vi "init runtime data structures.vi"(4 "write directory":path, 6 "read directory":path, 8 "error in":errorcluster, 9 "data allocations":T3, 10 "lines":T1[](array[typedef]), 11 "shared memory module runtime in":refnum<class "Shared Memory Runtime.lvclass">) -> (0 "error out":errorcluster, 3 "shared memory module runtime out":refnum<class "Shared Memory Runtime.lvclass">)   [LabVIEW 2013, in "Shared Memory Runtime.lvclass"]
uses:
  Shared Memory Runtime.lvclass
  <vilib>/NI/Tag Bus Module Framework/channel/data tables.ctl
  <vilib>/NI/Tag Bus/dictionary/data dictionary.lvclass
  <vilib>/NI/Tag Bus/dictionary table pair.ctl
  <vilib>/NI/Tag Bus/table/data table.ctl
  configuration/line configuration.ctl
  <vilib>/NI/Tag Bus Module Framework/channel/TBM channel.lvclass
  <vilib>/NI/Tag Bus/tag/Data Type.ctl
  <vilib>/NI/Tag Bus Module Framework/channel/channel classification.ctl
  <vilib>/NI/Tag Bus Module Framework/channel/TBM channel.lvclass/TBM channel.ctl
  <vilib>/NI/Tag Bus/tag/tag descriptor.lvclass/tag descriptor.ctl
  Shared Memory Runtime.lvclass/Shared Memory Runtime.ctl
  shared memory module runtime.ctl
  <vilib>/NI/Tag Bus/tag/read tag name.vi
  <vilib>/NI/Tag Bus/dictionary/locate tag.vi
  <vilib>/NI/Tag Bus/tag/tag descriptor.lvclass
  <vilib>/NI/Tag Bus/table/data table.lvlib
  <vilib>/NI/Tag Bus/tag bus.lvlib
  configuration/Shared Memory Configuration.lvclass
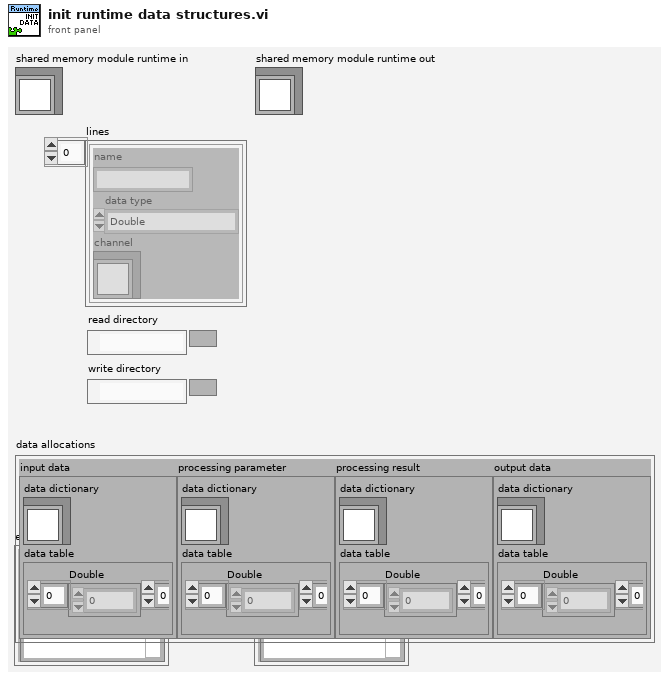
[diagram p1: front panel]
types:
  T1 = typedef "Shared Memory Configuration.lvclass/line configuration.ctl" = cluster{"name":string, "data type":T2, "channel":refnum<class "TBM channel.lvclass">}
  T2 = typedef "tag bus.lvlib/tag descriptor.lvclass/Data Type.ctl" = enum16{"Double", "Single", "I64", "I32", "I16", "I8", "U64", "U32", "U16", "U8", "Boolean", "String", "Array of Double", "Array of Single", "Array of I64", "Array of I32", "Array of I16", "Array of I8", "Array of U64", "Array of U32", "Array of U16", "Array of U8", "Array of Boolean", "Array of String"}
  T3 = typedef "TBM channel.lvclass/data tables.ctl" = cluster{"input data":T4, "processing parameter":T4, "processing result":T4, "output data":T4}
  T4 = typedef "tag bus.lvlib/dictionary table pair.ctl" = cluster{"data dictionary":refnum<class "data dictionary.lvclass">, "data table":T5}
  T5 = typedef "tag bus.lvlib/data table.lvlib/data table.ctl" = cluster{"Double":dbl[], "Single":sgl[], "I64":i64[], "I32":i32[], "I16":i16[], "I8":i8[], "U64":u64[], "U32":u32[], "U16":u16[], "U8":u8[], "Boolean":bool[], "String":string[], "Array of Double":cluster{"DBL Array":dbl[]}[], "Array of Single":cluster{"SGL Array":sgl[]}[], "Array of I64":cluster{"I64 Array":i64[]}[], "Array of I32":cluster{"I32 Array":i32[]}[], "Array of I16":cluster{"I16 Array":i16[]}[], "Array of I8":cluster{"I8 Array":i8[]}[], "Array of U64":cluster{"U64 Array":u64[]}[], "Array of U32":cluster{"U32 Array":u32[]}[], "Array of U16":cluster{"U16 Array":u16[]}[], "Array of U8":cluster{"U8 Array":u8[]}[], "Array of Boolean":cluster{"Boolean Array":bool[]}[], "Array of String":cluster{"String Array":string[]}[]}
  T6 = typedef "TBM channel.lvclass/channel classification.ctl" = enum16{"input data", "output data", "processing parameter", "processing result"}
  T7 = enum16{"open", "replace", "create", "open or create", "replace or create", "replace or create with confirmation"}
  T8 = typedef "Shared Memory Runtime.lvclass/shared memory module runtime.ctl" = cluster{"refnum":refnum<file>, "name":string, "data type":T2, "number of tags":i32, "indices":cluster{"index":i32[]}, "data array":cluster{"data":dbl[]}, "file array":cluster{"data":dbl[]}}
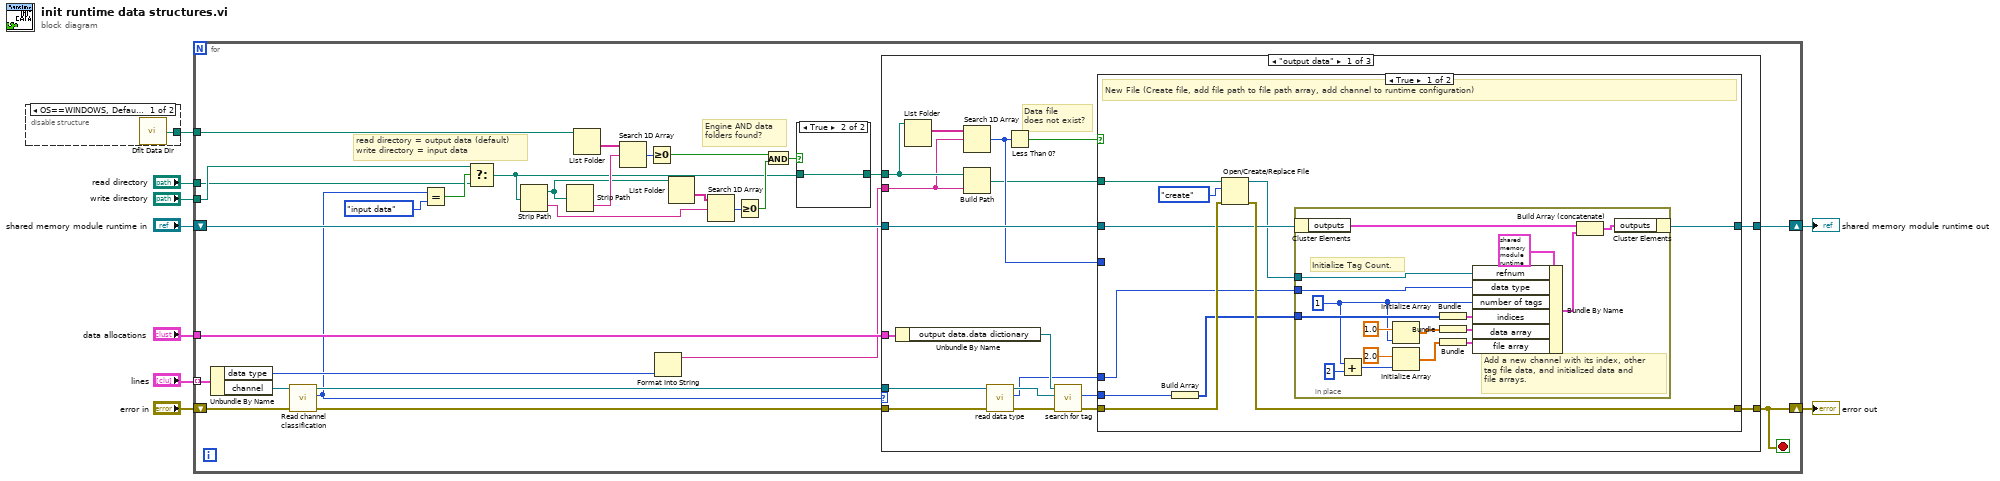
[diagram p0: block diagram]
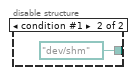
[diagram p2: hidden frame]
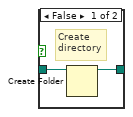
[diagram p3: hidden frame]
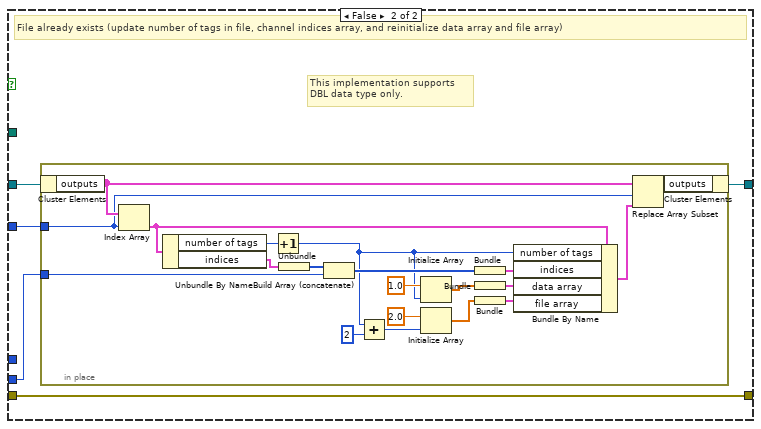
[diagram p4: hidden frame]
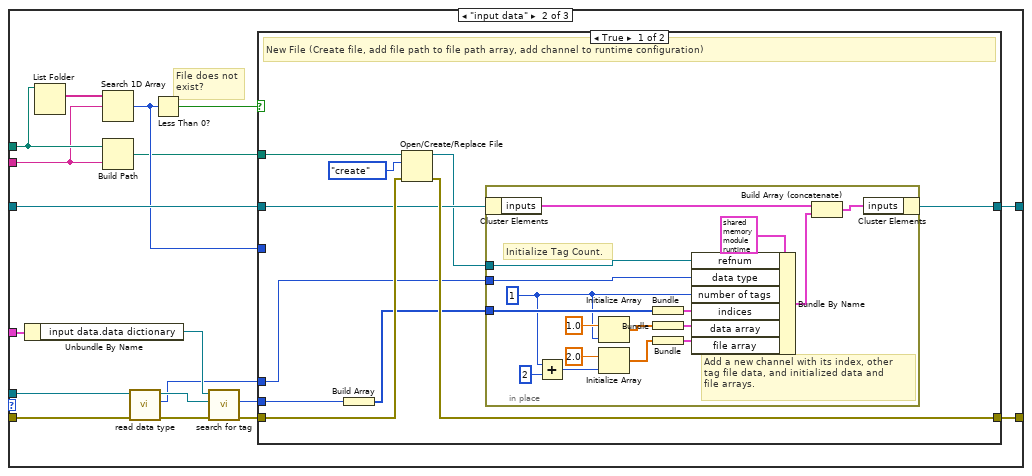
[diagram p5: hidden frame]
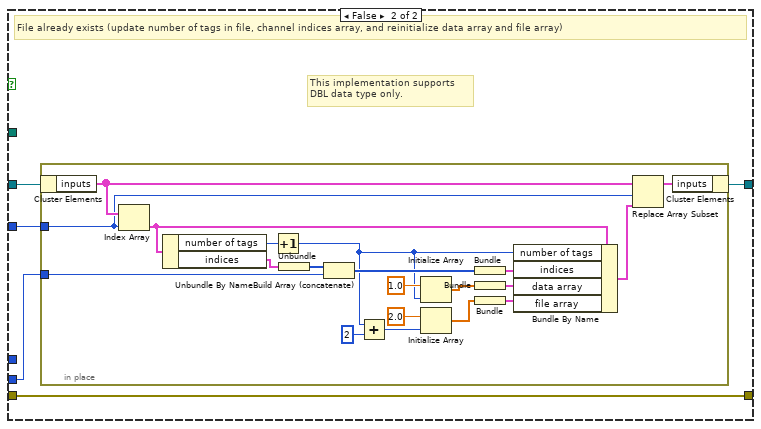
[diagram p6: hidden frame]
diagram:
  n1 = disable-structure shown="OS==WINDOWS, Default" {
    disable-tunnel: [w10 path "/dev/shm"] -> w3
    frame condition #0 (active) {
      n2 = call <vilib>:"Dflt Data Dir.vi"() -> ("App:Default Data Directory"=w10:path)
    }
    frame condition #1 {
    }
  }
  n3 = for {
    shift-right: [w40] -> w8
    shift-left: "error in" -> [w37]
    tunnel: "lines" -> [w38] mode=indexing
    tunnel: "data allocations" -> [w39]
    tunnel: w3 -> [w26]
    shift-right: [w32] -> w4
    shift-left: "shared memory module runtime in" -> [w33]
    tunnel: "read directory" -> [w12]
    tunnel: "write directory" -> [w13]
    stop <- w40 stop-if-true
    # "read directory = output data (default)\nwrite directory = input data"
    # "Engine AND data \nfolders found?"
    n4 = Unbundle By Name(w38) -> ("data type"=w31:T2, "channel"=w35:refnum<class "TBM channel.lvclass">)
    n5 = call <vilib>:"Read channel classification.vi"("error in"=w37, "channel in"=w35) -> ("error out"=w36:errorcluster, "channel classification"=w17:T6, "channel out"=w34:refnum<class "TBM channel.lvclass">)  [unwired: 7 in]
    n6 = Equal?(x=w17, y=channel_classification."input data") -> (x = y?=w15:bool)
    n7 = Select(t=w13, s=w15, f=w12) -> (s? t:f=w14:path)
    n8 = Strip Path(path=w14) -> (stripped path=w21:path, name=w19:string)
    n9 = Strip Path(path=w21) -> (name=w27:string)  [unwired: 1 out]
    n10 = List Folder(path=w26) -> (folder names=w29:string[])  [unwired: 3 in, 3 out]
    n11 = Search 1D Array(1D array=w29, element=w27) -> (index of element=w28:i32)  [unwired: 1 in]
    n12 = Greater Or Equal To 0?(x=w28) -> (x >= 0?=w24:bool)
    n13 = Format Into String(w31) -> (resulting string=w18:string)  [unwired: 3 in, 1 out]
    n14 = List Folder(path=w21) -> (folder names=w20:string[])  [unwired: 3 in, 3 out]
    n15 = Search 1D Array(1D array=w20, element=w19) -> (index of element=w25:i32)  [unwired: 1 in]
    n16 = Greater Or Equal To 0?(x=w25) -> (x >= 0?=w23:bool)
    n17 = And(x=w24, y=w23) -> (x .and. y?=w22:bool)
    n18 = case shown="True" w22 {
      tunnel: [w41 w43] -> w30
      tunnel: w14 -> [w42 w43]
      frame False {
        # "Create\ndirectory"
        n19 = Create Folder(path (use dialog)=w42) -> (created path=w41:path)  [unwired: 2 in, 2 out]
      }
      frame True {
      }
    }
    n20 = case shown="\"output data\"" w17 {
      tunnel: [w53 w123 w185] -> w40
      tunnel: w36 -> [w60 w130 w185]
      tunnel: w39 -> [w58 w128 _]
      tunnel: w34 -> [w56 w126 _]
      tunnel: w30 -> [w46 w116 _]
      tunnel: w18 -> [w45 w115 _]
      tunnel: w33 -> [w51 w121 w184]
      tunnel: [w50 w120 w184] -> w32
      frame "output data" {
        # "Data file \ndoes not exist?"
        n21 = Unbundle By Name(w58) -> ("output data.data dictionary"=w57:refnum<class "data dictionary.lvclass">)
        n22 = List Folder(path=w46) -> (filenames=w47:string[])  [unwired: 3 in, 3 out]
        n23 = Search 1D Array(1D array=w47, element=w45) -> (index of element=w49:i32)  [unwired: 1 in]
        n24 = Build Path(base path=w46, name or relative path=w45) -> (appended path=w44:path)
        n25 = call <vilib>:"read data type.vi"("error in"=w60, "system tag in"=w56) -> ("error out"=w59:errorcluster, "data type"=w54:T2, "system tag out"=w61:refnum<class "TBM channel.lvclass">)  [unwired: 7 in]
        n26 = Less Than 0?(x=w49) -> (x < 0?=w52:bool)
        n27 = call <vilib>:"search for tag.vi"("error in"=w59, "system tag"=w61, "data dictionary in"=w57) -> ("error out"=w55:errorcluster, "index"=w48:i32)  [unwired: 6 in, 1 out]
        n28 = case shown="True" w52 {
          tunnel: w44 -> [w69 _]
          tunnel: w55 -> [w71 w93]
          tunnel: w54 -> [w64 _]
          tunnel: [w70 w93] -> w53
          tunnel: w51 -> [w67 w92]
          tunnel: [w66 w90] -> w50
          tunnel: w49 -> [_ w91]
          tunnel: w48 -> [w63 w89]
          frame True {
            # "New File (Create file, add file path to file path array, add channel to runtime configuration)"
            n29 = Build Array(w63) -> (w62:i32[])
            n30 = Open/Create/Replace File(file path (use dialog)=w69, error in=w71, operation (0:open)=T7."create") -> (refnum out=w65:refnum<file>, error out=w70:errorcluster)  [unwired: 3 in, 1 out]
            n31 = in-place {
              in-place-border: w62 -> [w88]
              in-place-border: w65 -> [w78]
              in-place-border: w64 -> [w77]
              w72 = 1 ("y")
              # "Initialize Tag Count."
              # "Add a new channel with its index, other \ntag file data, and initialized data and \nfile arrays."
              n32 = in-place-cluster #1(w67) -> ("outputs"=w76:T8[])
              n33 = Add(x=w72, y=2) -> (x+y=w79:i32)
              n34 = Initialize Array(1.0 ("element"), w72) -> (w84:dbl[])
              n35 = Initialize Array(2.0 ("element"), w79) -> (w82:dbl[])
              n36 = Bundle(w88) -> (w87:cluster{i32[]})  [unwired: 1 in]
              n37 = Bundle(w84) -> (w83:cluster{dbl[]})  [unwired: 1 in]
              n38 = Bundle(w82) -> (w81:cluster{dbl[]})  [unwired: 1 in]
              n39 = Bundle By Name(cluster=T8 {"refnum"=refnum, "name"="", "data type"=enum."Double", "number of tags"=0, "indices"={"index"=[]}, "data array"={"data"=[]}, "file array"={"data"=[]}} ("tag config"), "refnum"=w78, "data type"=w77, "number of tags"=w72, "indices"=w87, "data array"=w83, "file array"=w81) -> (w73:T8)
              n40 = Build Array (concatenate)(w76, w73) -> (w75:T8[])
              n41 = in-place-cluster #1("outputs"=w75) -> (w66:refnum<class "Shared Memory Runtime.lvclass">)
            }
          }
          frame False {
            # "This implementation supports \nDBL data type only."
            # "File already exists (update number of tags in file, channel indices array, and reinitialize data array and file array)"
            n42 = in-place {
              in-place-border: w91 -> [w101]
              in-place-border: w89 -> [w97]
              n43 = in-place-cluster #2(w92) -> ("outputs"=w104:T8[])
              n44 = Index Array(array=w104, index=w101) -> (element=w100:T8)
              n45 = Unbundle By Name(w100) -> ("number of tags"=w95:i32, "indices"=w99:cluster{"index":i32[]})
              n46 = Increment(x=w95) -> (x+1=w94:i32)
              n47 = Unbundle(w99) -> ("index"=w98:i32[])
              n48 = Build Array (concatenate)(w98, w97) -> (w96:i32[])
              n49 = Add(x=w94, y=2) -> (x+y=w105:i32)
              n50 = Initialize Array(1.0 ("element"), w94) -> (w110:dbl[])
              n51 = Initialize Array(2.0 ("element"), w105) -> (w108:dbl[])
              n52 = Bundle(w96) -> (w113:cluster{i32[]})  [unwired: 1 in]
              n53 = Bundle(w110) -> (w109:cluster{dbl[]})  [unwired: 1 in]
              n54 = Bundle(w108) -> (w107:cluster{dbl[]})  [unwired: 1 in]
              n55 = Bundle By Name(cluster=w100, "number of tags"=w94, "indices"=w113, "data array"=w109, "file array"=w107) -> (w102:T8)
              n56 = Replace Array Subset(array=w104, new element=w102, index=w101) -> (w103:T8[])
              n57 = in-place-cluster #2("outputs"=w103) -> (w90:refnum<class "Shared Memory Runtime.lvclass">)
            }
          }
        }
      }
      frame "input data" {
        # "File does not\nexist?"
        n58 = Unbundle By Name(w128) -> ("input data.data dictionary"=w127:refnum<class "data dictionary.lvclass">)
        n59 = List Folder(path=w116) -> (filenames=w117:string[])  [unwired: 3 in, 3 out]
        n60 = Search 1D Array(1D array=w117, element=w115) -> (index of element=w119:i32)  [unwired: 1 in]
        n61 = Build Path(base path=w116, name or relative path=w115) -> (appended path=w114:path)
        n62 = call <vilib>:"read data type.vi"("error in"=w130, "system tag in"=w126) -> ("error out"=w129:errorcluster, "data type"=w124:T2, "system tag out"=w131:refnum<class "TBM channel.lvclass">)  [unwired: 7 in]
        n63 = Less Than 0?(x=w119) -> (x < 0?=w122:bool)
        n64 = call <vilib>:"search for tag.vi"("error in"=w129, "system tag"=w131, "data dictionary in"=w127) -> ("error out"=w125:errorcluster, "index"=w118:i32)  [unwired: 6 in, 1 out]
        n65 = case shown="True" w122 {
          tunnel: w114 -> [w139 _]
          tunnel: w125 -> [w141 w163]
          tunnel: w124 -> [w134 _]
          tunnel: [w140 w163] -> w123
          tunnel: w121 -> [w137 w162]
          tunnel: [w136 w160] -> w120
          tunnel: w119 -> [_ w161]
          tunnel: w118 -> [w133 w159]
          frame True {
            # "New File (Create file, add file path to file path array, add channel to runtime configuration)"
            n66 = Build Array(w133) -> (w132:i32[])
            n67 = Open/Create/Replace File(file path (use dialog)=w139, error in=w141, operation (0:open)=T7."create") -> (refnum out=w135:refnum<file>, error out=w140:errorcluster)  [unwired: 3 in, 1 out]
            n68 = in-place {
              in-place-border: w132 -> [w158]
              in-place-border: w135 -> [w148]
              in-place-border: w134 -> [w147]
              w142 = 1 ("y")
              # "Initialize Tag Count."
              # "Add a new channel with its index, other \ntag file data, and initialized data and \nfile arrays."
              n69 = in-place-cluster #3(w137) -> ("inputs"=w146:T8[])
              n70 = Add(x=w142, y=2) -> (x+y=w149:i32)
              n71 = Initialize Array(1.0 ("element"), w142) -> (w154:dbl[])
              n72 = Initialize Array(2.0 ("element"), w149) -> (w152:dbl[])
              n73 = Bundle(w158) -> (w157:cluster{i32[]})  [unwired: 1 in]
              n74 = Bundle(w154) -> (w153:cluster{dbl[]})  [unwired: 1 in]
              n75 = Bundle(w152) -> (w151:cluster{dbl[]})  [unwired: 1 in]
              n76 = Bundle By Name(cluster=T8 {"refnum"=refnum, "name"="", "data type"=enum."Double", "number of tags"=0, "indices"={"index"=[]}, "data array"={"data"=[]}, "file array"={"data"=[]}} ("tag config"), "refnum"=w148, "data type"=w147, "number of tags"=w142, "indices"=w157, "data array"=w153, "file array"=w151) -> (w143:T8)
              n77 = Build Array (concatenate)(w146, w143) -> (w145:T8[])
              n78 = in-place-cluster #3("inputs"=w145) -> (w136:refnum<class "Shared Memory Runtime.lvclass">)
            }
          }
          frame False {
            # "This implementation supports \nDBL data type only."
            # "File already exists (update number of tags in file, channel indices array, and reinitialize data array and file array)"
            n79 = in-place {
              in-place-border: w161 -> [w171]
              in-place-border: w159 -> [w167]
              n80 = in-place-cluster #4(w162) -> ("inputs"=w174:T8[])
              n81 = Index Array(array=w174, index=w171) -> (element=w170:T8)
              n82 = Unbundle By Name(w170) -> ("number of tags"=w165:i32, "indices"=w169:cluster{"index":i32[]})
              n83 = Increment(x=w165) -> (x+1=w164:i32)
              n84 = Unbundle(w169) -> ("index"=w168:i32[])
              n85 = Build Array (concatenate)(w168, w167) -> (w166:i32[])
              n86 = Add(x=w164, y=2) -> (x+y=w175:i32)
              n87 = Initialize Array(1.0 ("element"), w164) -> (w180:dbl[])
              n88 = Initialize Array(2.0 ("element"), w175) -> (w178:dbl[])
              n89 = Bundle(w166) -> (w183:cluster{i32[]})  [unwired: 1 in]
              n90 = Bundle(w180) -> (w179:cluster{dbl[]})  [unwired: 1 in]
              n91 = Bundle(w178) -> (w177:cluster{dbl[]})  [unwired: 1 in]
              n92 = Bundle By Name(cluster=w170, "number of tags"=w164, "indices"=w183, "data array"=w179, "file array"=w177) -> (w172:T8)
              n93 = Replace Array Subset(array=w174, new element=w172, index=w171) -> (w173:T8[])
              n94 = in-place-cluster #4("inputs"=w173) -> (w160:refnum<class "Shared Memory Runtime.lvclass">)
            }
          }
        }
      }
      frame Default {
        # "Tag is not an input or output channel."
      }
    }
  }
  "shared memory module runtime out" <- w4
  "error out" <- w8
